vi "生成报告.vi"(6 "目标温度":string(combo), 7 "样品编号":string, 8 "均匀性表格":string[][](table)=[["A", "O", "E", "O"], ["", "", "", ""], ["", "", "", ""], ["", "", "", ""], ["", "", "", ""], ["", "", "", ""], ["", "", "", ""], ["B", "O", "F", "O"], ["", "", "", ""], ["", "", "", ""], ["", "", "", ""], ["", "", "", ""], ["", "", "", ""], ["", "", "", ""], ["C", "O", "G", "O"], ["", "", "", ""], ["", "", "", ""], ["", "", "", ""], ["", "", "", ""], ["", "", "", ""], ["", "", "", ""], ["D", "O", "H", "O"], ["", "", "", ""], ["", "", "", ""], ["", "", "", ""], ["", "", "", ""], ["", "", "", ""], ["", "", "", ""], ["", "", "", ""], ["", "", "", ""]], 10 "波动性表格":string[][](table), 11 "原始记录路径":path caption="模板（空）") -> ()   [LabVIEW 2015]
uses:
  <vilib>/addons/_office/_exclsub.llb/font.ctl
  <vilib>/addons/_office/excel.llb/Excel Easy Table (str).vi
  <vilib>/Utility/NIReport.llb/NI_report.lvclass
  <vilib>/addons/_office/NI_ReportGenerationToolkit.lvlib
  <vilib>/Utility/NIReport.llb/Excel/NI_Excel.lvclass
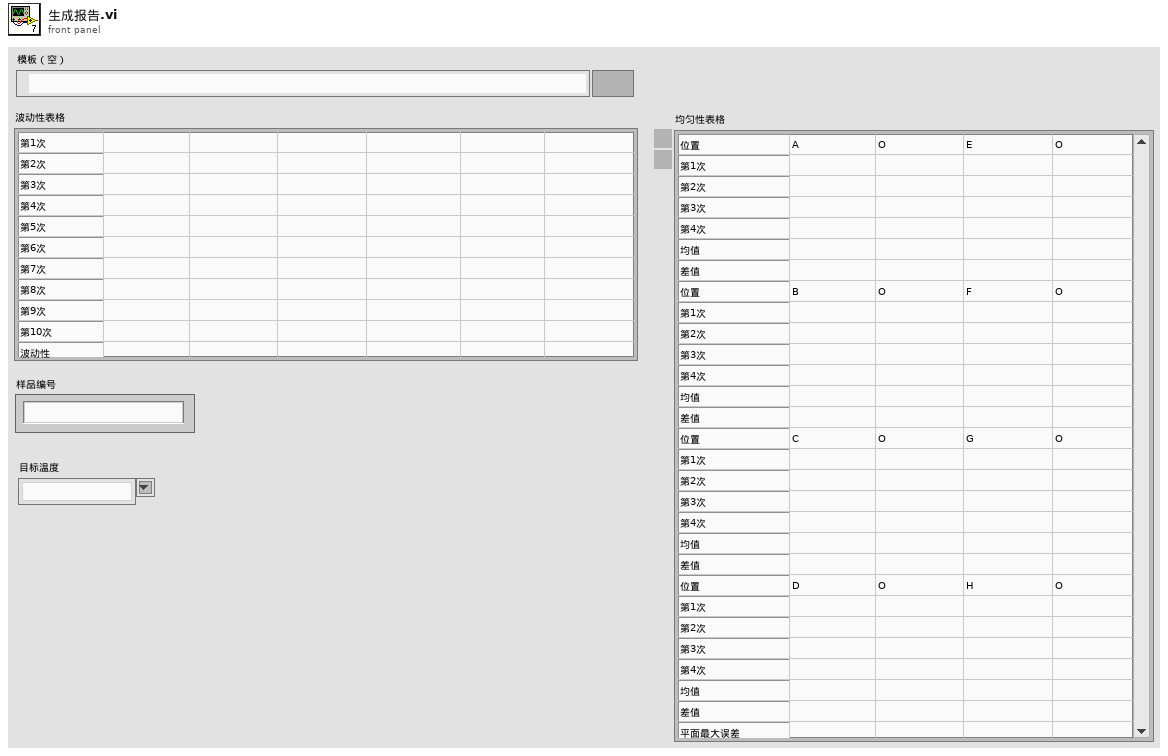
[diagram p1: front panel]
types:
  T1 = typedef "NI_ReportGenerationToolkit.lvlib/font.ctl" = cluster{"font name":string, "font size":dbl, "bold":u16, "italic":u16, "underline":u16, "strike through":u16, "font color":u32}
  T2 = enum16{"maximized", "minimized", "normal", "no change"}
  T3 = enum16{"Standard Report", "HTML", "Word", "Excel"}
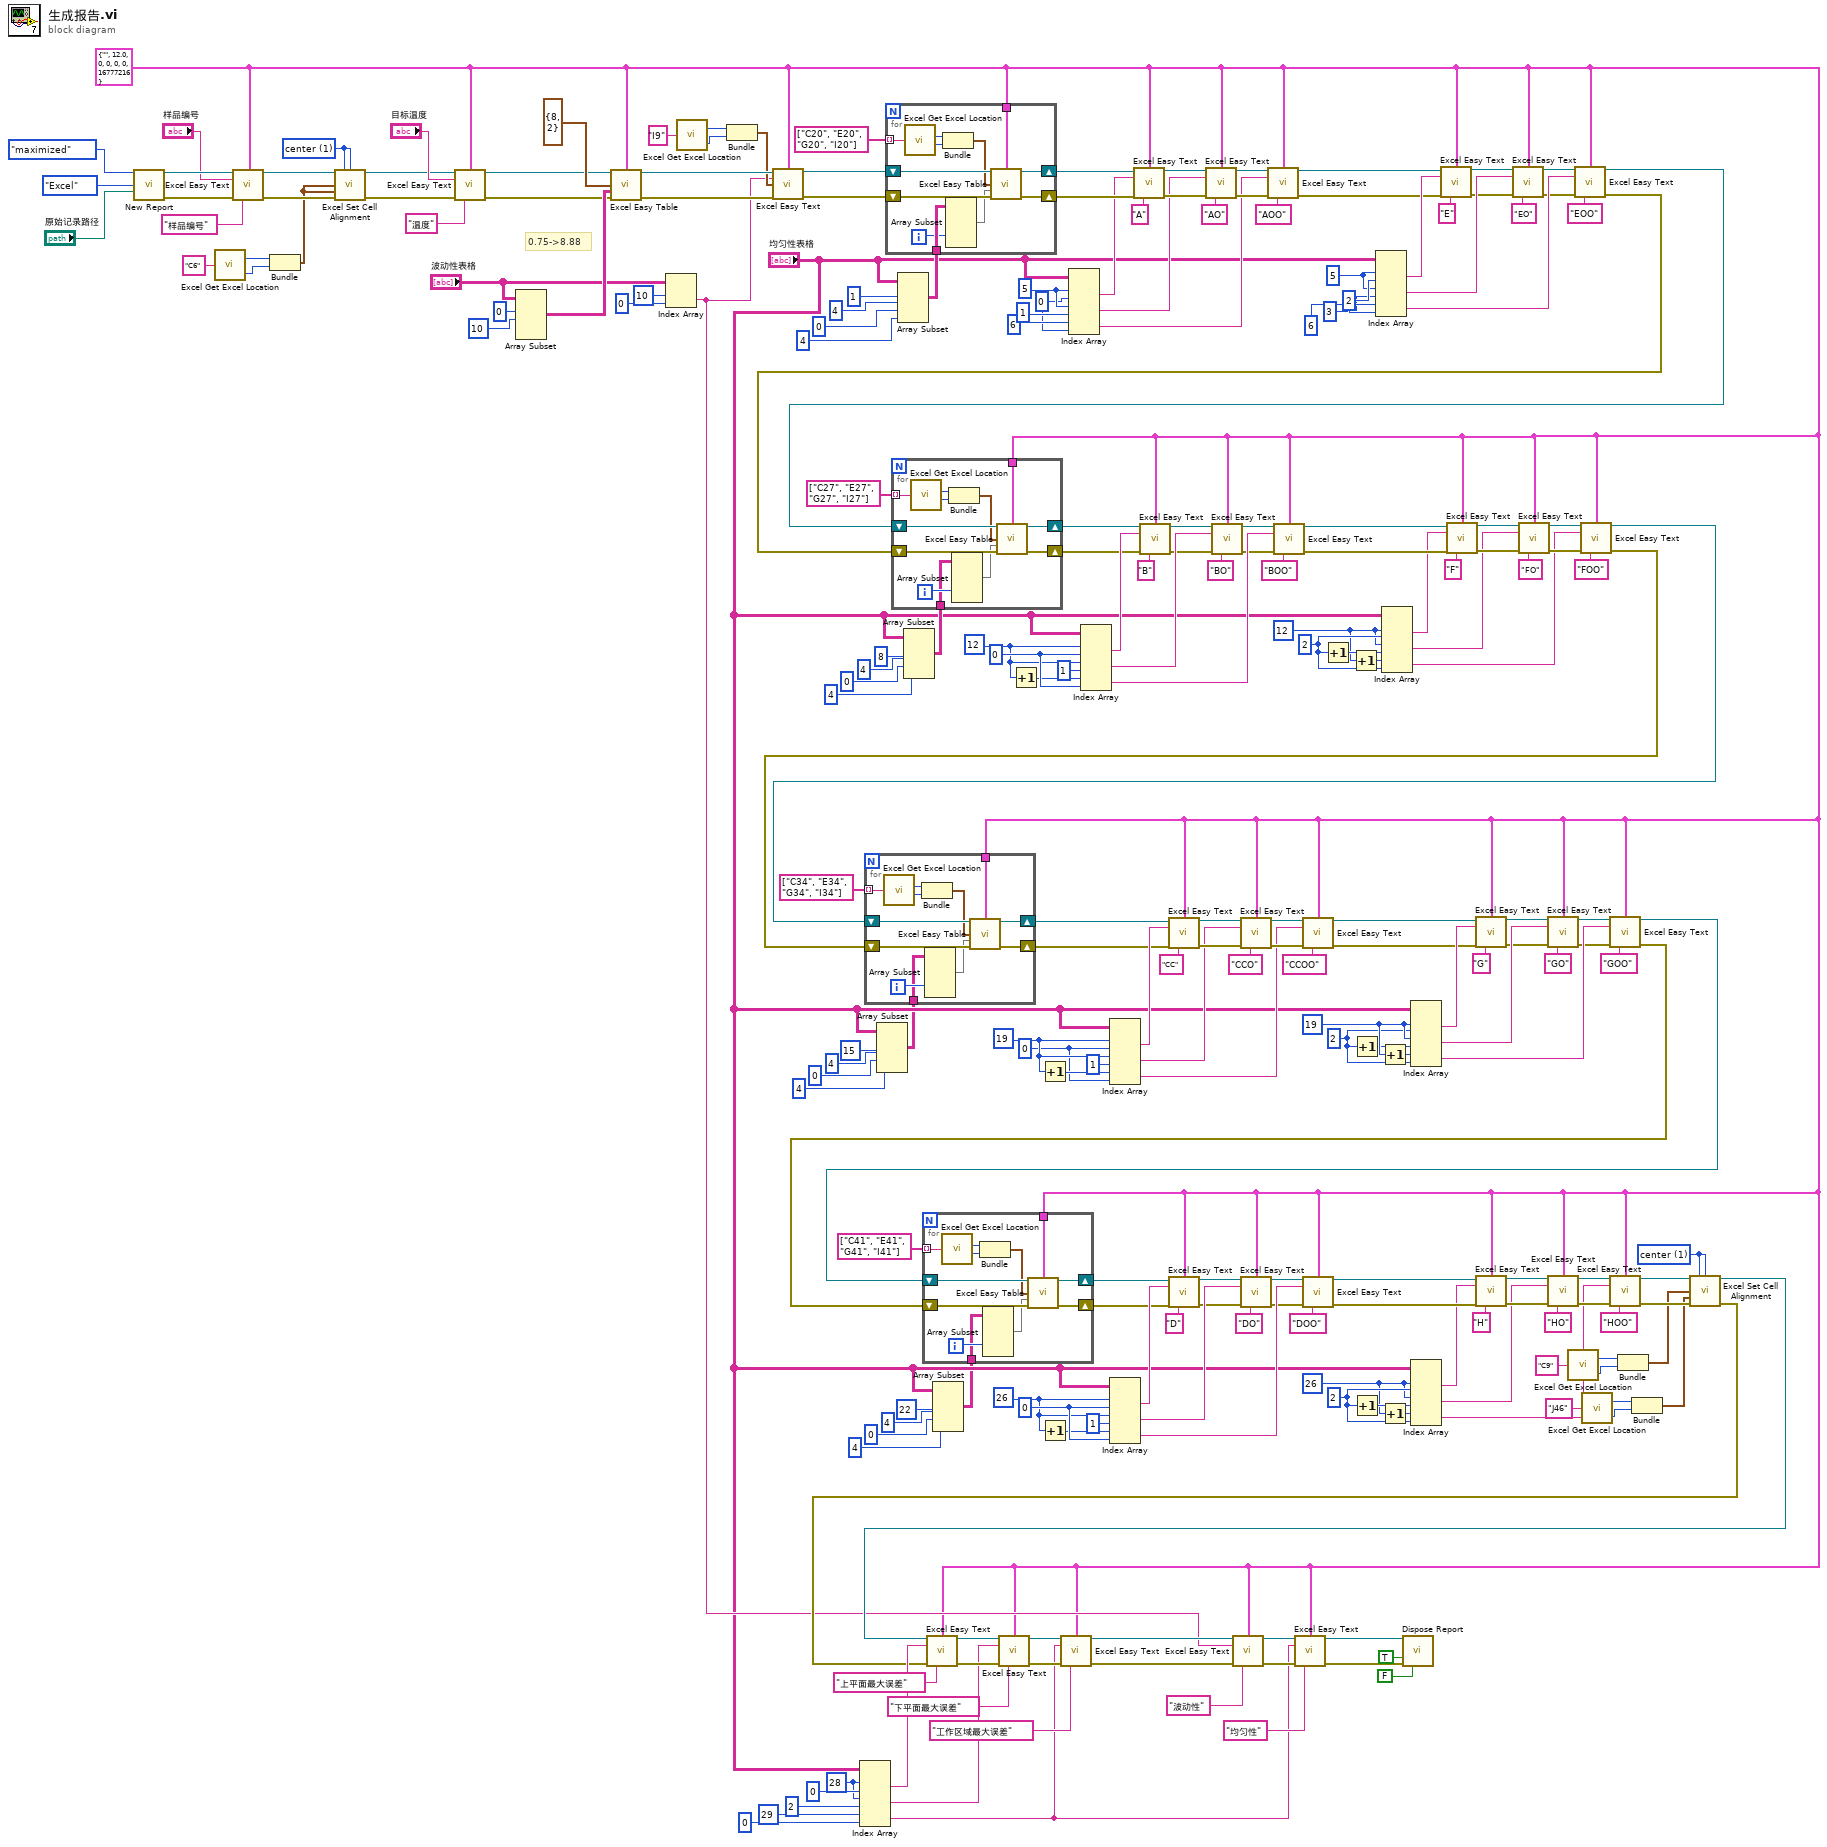
[diagram p0: block diagram]
diagram:
  w30 = 1 items=["top", "center", "bottom"] ("vertical alignment (top)")
  w59 = 1 items=["top", "center", "bottom"] ("vertical alignment (top)")
  w68 = 28 ("索引")
  w81 = 2 ("索引")
  w79 = 26 ("长度")
  w99 = 0 ("索引")
  w83 = 26 ("长度")
  w142 = 2 ("索引")
  w144 = 19 ("长度")
  w124 = 0 ("索引")
  w140 = 19 ("长度")
  w149 = 2 ("索引")
  w147 = 12 ("长度")
  w167 = 0 ("索引")
  w151 = 12 ("长度")
  w3 = T1 {"font name"="", "font size"=12.0, "bold"=0, "italic"=0, "underline"=0, "strike through"=0, "font color"=16777216} ("font")
  w195 = 2 ("索引")
  w192 = 5 ("长度")
  w196 = 0 ("索引")
  w199 = 5 ("长度")
  # "0.75->8.88"
  n1 = call <vilib>:"New Report.vi"("window state (normal)"=T2."maximized", "report type"=T3."Excel", "template (empty)"="原始记录路径") -> ("report out"=w37:refnum<class "NI_report.lvclass">, "error out"=w38:errorcluster)  [unwired: 11 in]
  n2 = call <vilib>:"Excel Get Excel Location.vi"("cell's name"="C6") -> ("row"=w23:i32, "column"=w24:i32)
  n3 = call <vilib>:"Excel Easy Text.vi"("report in"=w37, "font"=w3, "text"="样品编号", "error in (no error)"=w38, "name (\"\")"="样品编号" ("name (\"\")")) -> ("report out"=w27:refnum<class "NI_report.lvclass">, "error out"=w29:errorcluster)  [unwired: 6 in, 3 out]
  n4 = Bundle("row"=w23, "column"=w24) -> (w22:cluster{"row":i32, "column":i32})  [unwired: 1 in]
  n5 = call <vilib>:"Excel Set Cell Alignment.vi"("report in"=w27, "vertical alignment (top)"=w30, "horizontal alignment (left)"=w30, "start (-1, -1)"=w22, "end (-1, -1)"=w22, "error in (no error)"=w29) -> ("report out"=w26:refnum<class "NI_report.lvclass">, "error out"=w28:errorcluster)  [unwired: 8 in]
  n6 = call <vilib>:"Excel Easy Text.vi"("report in"=w26, "font"=w3, "text"="目标温度", "error in (no error)"=w28, "name (\"\")"="温度" ("name (\"\")")) -> ("report out"=w35:refnum<class "NI_report.lvclass">, "error out"=w36:errorcluster)  [unwired: 6 in, 3 out]
  n7 = Array Subset(array="波动性表格", index (row)=0 ("索引"), length (row)=10 ("索引")) -> (w228:string[][])  [unwired: 2 in]
  n8 = call-poly <vilib>:"Excel Easy Table.vi"("report in"=w35, "font"=w3, "start (0, 0)"=cluster{"row":i32, "column":i32} {"row"=8, "column"=2}, "text data"=w228, "error in (no error)"=w36) -> ("report out"=w224:refnum<class "NI_report.lvclass">, "error out"=w223:errorcluster)  [unwired: 6 in, 3 out]
  n9 = Index Array(array="波动性表格", index (row)=10 ("索引 (行)"), index (col)=0 ("索引 (行)")) -> (element=w43:string)
  n10 = call <vilib>:"Excel Get Excel Location.vi"("cell's name"="I9") -> ("row"=w220:i32, "column"=w221:i32)
  n11 = Bundle("row"=w220, "column"=w221) -> (w219:cluster{"row":i32, "column":i32})  [unwired: 1 in]
  n12 = call <vilib>:"Excel Easy Text.vi"("report in"=w224, "font"=w3, "text"=w43, "start (-1, -1)"=w219, "error in (no error)"=w223) -> ("report out"=w218:refnum<class "NI_report.lvclass">, "error out"=w217:errorcluster)  [unwired: 6 in, 3 out]
  n13 = Index Array(array="均匀性表格", index (row) #1=w68, index (col) #1=0 ("索引"), index (row) #2=w68, index (col) #2=2 ("长度"), index (row) #3=29 ("索引"), index (col) #3=0 ("索引")) -> (element #1=w70:string, element #2=w64:string, element #3=w44:string)
  n14 = Array Subset(array="均匀性表格", index (row)=15 ("索引"), length (row)=4 ("长度"), index (col)=0 ("索引"), length (col)=4 ("索引")) -> (w1:string[][])
  n15 = Array Subset(array="均匀性表格", index (row)=1 ("索引"), length (row)=4 ("长度"), index (col)=0 ("索引"), length (col)=4 ("索引")) -> (w212:string[][])
  n16 = for {
    tunnel: w212 -> [w237]
    tunnel: w3 -> [w239]
    shift-right: [w240] -> w210
    shift-left: w218 -> [w246]
    shift-right: [w241] -> w211
    shift-left: w217 -> [w245]
    tunnel: string[] ["C20", "E20", "G20", "I20"] -> [w238] mode=indexing
    i -> [w235]
    n17 = call <vilib>:"Excel Get Excel Location.vi"("cell's name"=w238) -> ("row"=w244:i32, "column"=w243:i32)
    n18 = Bundle("row"=w244, "column"=w243) -> (w242:cluster{"row":i32, "column":i32})  [unwired: 1 in]
    n19 = Array Subset(array=w237, index (col)=w235) -> (w236:string[][])  [unwired: 3 in]
    n20 = call-poly <vilib>:"Excel Easy Table.vi"("report in"=w246, "font"=w239, "start (0, 0)"=w242, "text data"=w236, "error in (no error)"=w245) -> ("report out"=w240:refnum<class "NI_report.lvclass">, "error out"=w241:errorcluster)  [unwired: 6 in, 3 out]
  }
  n21 = Array Subset(array="均匀性表格", index (row)=8 ("索引"), length (row)=4 ("长度"), index (col)=0 ("索引"), length (col)=4 ("索引")) -> (w15:string[][])
  n22 = Array Subset(array="均匀性表格", index (row)=22 ("索引"), length (row)=4 ("长度"), index (col)=0 ("索引"), length (col)=4 ("索引")) -> (w2:string[][])
  n23 = Increment(x=w151) -> (x+1=w150:i32)
  n24 = Increment(x=w140) -> (x+1=w141:i32)
  n25 = Increment(x=w83) -> (x+1=w82:i32)
  n26 = Index Array(array="均匀性表格", index (row) #1=w199, index (col) #1=w196, index (row) #2=w199, index (col) #2=1 ("索引"), index (row) #3=6 ("长度"), index (col) #3=w196) -> (element #1=w209:string, element #2=w201:string, element #3=w200:string)
  n27 = Index Array(array="均匀性表格", index (row) #1=w151, index (col) #1=w167, index (row) #2=w151, index (col) #2=1 ("索引"), index (row) #3=w150, index (col) #3=w167) -> (element #1=w156:string, element #2=w164:string, element #3=w165:string)
  n28 = Index Array(array="均匀性表格", index (row) #1=w140, index (col) #1=w124, index (row) #2=w140, index (col) #2=1 ("索引"), index (row) #3=w141, index (col) #3=w124) -> (element #1=w135:string, element #2=w127:string, element #3=w126:string)
  n29 = Index Array(array="均匀性表格", index (row) #1=w83, index (col) #1=w99, index (row) #2=w83, index (col) #2=1 ("索引"), index (row) #3=w82, index (col) #3=w99) -> (element #1=w88:string, element #2=w96:string, element #3=w97:string)
  n30 = call <vilib>:"Excel Easy Text.vi"("report in"=w210, "font"=w3, "text"=w209, "error in (no error)"=w211, "name (\"\")"="A" ("name (\"\")")) -> ("report out"=w207:refnum<class "NI_report.lvclass">, "error out"=w206:errorcluster)  [unwired: 6 in, 3 out]
  n31 = call <vilib>:"Excel Easy Text.vi"("report in"=w207, "font"=w3, "text"=w201, "error in (no error)"=w206, "name (\"\")"="AO" ("name (\"\")")) -> ("report out"=w203:refnum<class "NI_report.lvclass">, "error out"=w202:errorcluster)  [unwired: 6 in, 3 out]
  n32 = call <vilib>:"Excel Easy Text.vi"("report in"=w203, "font"=w3, "text"=w200, "error in (no error)"=w202, "name (\"\")"="AOO" ("name (\"\")")) -> ("report out"=w180:refnum<class "NI_report.lvclass">, "error out"=w181:errorcluster)  [unwired: 6 in, 3 out]
  n33 = Increment(x=w149) -> (x+1=w148:i32)
  n34 = Increment(x=w147) -> (x+1=w146:i32)
  n35 = Increment(x=w142) -> (x+1=w143:i32)
  n36 = Increment(x=w81) -> (x+1=w80:i32)
  n37 = Index Array(array="均匀性表格", index (row) #1=w192, index (col) #1=w195, index (row) #2=w192, index (col) #2=3 ("索引"), index (row) #3=6 ("长度"), index (col) #3=w195) -> (element #1=w182:string, element #2=w190:string, element #3=w191:string)
  n38 = Increment(x=w144) -> (x+1=w145:i32)
  n39 = Increment(x=w79) -> (x+1=w78:i32)
  n40 = Index Array(array="均匀性表格", index (row) #1=w147, index (col) #1=w149, index (row) #2=w147, index (col) #2=w148, index (row) #3=w146, index (col) #3=w149) -> (element #1=w177:string, element #2=w169:string, element #3=w168:string)
  n41 = Index Array(array="均匀性表格", index (row) #1=w144, index (col) #1=w142, index (row) #2=w144, index (col) #2=w143, index (row) #3=w145, index (col) #3=w142) -> (element #1=w114:string, element #2=w122:string, element #3=w123:string)
  n42 = Index Array(array="均匀性表格", index (row) #1=w79, index (col) #1=w81, index (row) #2=w79, index (col) #2=w80, index (row) #3=w78, index (col) #3=w81) -> (element #1=w109:string, element #2=w101:string, element #3=w100:string)
  n43 = call <vilib>:"Excel Easy Text.vi"("report in"=w180, "font"=w3, "text"=w182, "error in (no error)"=w181, "name (\"\")"="E" ("name (\"\")")) -> ("report out"=w184:refnum<class "NI_report.lvclass">, "error out"=w185:errorcluster)  [unwired: 6 in, 3 out]
  n44 = call <vilib>:"Excel Easy Text.vi"("report in"=w184, "font"=w3, "text"=w190, "error in (no error)"=w185, "name (\"\")"="EO" ("name (\"\")")) -> ("report out"=w188:refnum<class "NI_report.lvclass">, "error out"=w189:errorcluster)  [unwired: 6 in, 3 out]
  n45 = call <vilib>:"Excel Get Excel Location.vi"("cell's name"="C9") -> ("row"=w56:i32, "column"=w57:i32)
  n46 = call <vilib>:"Excel Easy Text.vi"("report in"=w188, "font"=w3, "text"=w191, "error in (no error)"=w189, "name (\"\")"="EOO" ("name (\"\")")) -> ("report out"=w20:refnum<class "NI_report.lvclass">, "error out"=w19:errorcluster)  [unwired: 6 in, 3 out]
  n47 = for {
    tunnel: w15 -> [w247]
    tunnel: w3 -> [w251]
    shift-right: [w252] -> w18
    shift-left: w20 -> [w258]
    shift-right: [w253] -> w17
    shift-left: w19 -> [w257]
    tunnel: string[] ["C27", "E27", "G27", "I27"] -> [w250] mode=indexing
    i -> [w248]
    n48 = call <vilib>:"Excel Get Excel Location.vi"("cell's name"=w250) -> ("row"=w256:i32, "column"=w255:i32)
    n49 = Bundle("row"=w256, "column"=w255) -> (w254:cluster{"row":i32, "column":i32})  [unwired: 1 in]
    n50 = Array Subset(array=w247, index (col)=w248) -> (w249:string[][])  [unwired: 3 in]
    n51 = call-poly <vilib>:"Excel Easy Table.vi"("report in"=w258, "font"=w251, "start (0, 0)"=w254, "text data"=w249, "error in (no error)"=w257) -> ("report out"=w252:refnum<class "NI_report.lvclass">, "error out"=w253:errorcluster)  [unwired: 6 in, 3 out]
  }
  n52 = call <vilib>:"Excel Easy Text.vi"("report in"=w18, "font"=w3, "text"=w156, "error in (no error)"=w17, "name (\"\")"="B" ("name (\"\")")) -> ("report out"=w158:refnum<class "NI_report.lvclass">, "error out"=w159:errorcluster)  [unwired: 6 in, 3 out]
  n53 = call <vilib>:"Excel Easy Text.vi"("report in"=w158, "font"=w3, "text"=w164, "error in (no error)"=w159, "name (\"\")"="BO" ("name (\"\")")) -> ("report out"=w162:refnum<class "NI_report.lvclass">, "error out"=w163:errorcluster)  [unwired: 6 in, 3 out]
  n54 = call <vilib>:"Excel Easy Text.vi"("report in"=w162, "font"=w3, "text"=w165, "error in (no error)"=w163, "name (\"\")"="BOO" ("name (\"\")")) -> ("report out"=w179:refnum<class "NI_report.lvclass">, "error out"=w178:errorcluster)  [unwired: 6 in, 3 out]
  n55 = call <vilib>:"Excel Easy Text.vi"("report in"=w179, "font"=w3, "text"=w177, "error in (no error)"=w178, "name (\"\")"="F" ("name (\"\")")) -> ("report out"=w175:refnum<class "NI_report.lvclass">, "error out"=w174:errorcluster)  [unwired: 6 in, 3 out]
  n56 = call <vilib>:"Excel Easy Text.vi"("report in"=w175, "font"=w3, "text"=w169, "error in (no error)"=w174, "name (\"\")"="FO" ("name (\"\")")) -> ("report out"=w171:refnum<class "NI_report.lvclass">, "error out"=w170:errorcluster)  [unwired: 6 in, 3 out]
  n57 = call <vilib>:"Excel Easy Text.vi"("report in"=w171, "font"=w3, "text"=w168, "error in (no error)"=w170, "name (\"\")"="FOO" ("name (\"\")")) -> ("report out"=w10:refnum<class "NI_report.lvclass">, "error out"=w9:errorcluster)  [unwired: 6 in, 3 out]
  n58 = for {
    tunnel: w1 -> [w259]
    tunnel: w3 -> [w263]
    shift-right: [w264] -> w12
    shift-left: w10 -> [w270]
    shift-right: [w265] -> w13
    shift-left: w9 -> [w269]
    tunnel: string[] ["C34", "E34", "G34", "I34"] -> [w262] mode=indexing
    i -> [w260]
    n59 = call <vilib>:"Excel Get Excel Location.vi"("cell's name"=w262) -> ("row"=w268:i32, "column"=w267:i32)
    n60 = Bundle("row"=w268, "column"=w267) -> (w266:cluster{"row":i32, "column":i32})  [unwired: 1 in]
    n61 = Array Subset(array=w259, index (col)=w260) -> (w261:string[][])  [unwired: 3 in]
    n62 = call-poly <vilib>:"Excel Easy Table.vi"("report in"=w270, "font"=w263, "start (0, 0)"=w266, "text data"=w261, "error in (no error)"=w269) -> ("report out"=w264:refnum<class "NI_report.lvclass">, "error out"=w265:errorcluster)  [unwired: 6 in, 3 out]
  }
  n63 = call <vilib>:"Excel Easy Text.vi"("report in"=w12, "font"=w3, "text"=w135, "error in (no error)"=w13, "name (\"\")"="CC" ("name (\"\")")) -> ("report out"=w133:refnum<class "NI_report.lvclass">, "error out"=w132:errorcluster)  [unwired: 6 in, 3 out]
  n64 = call <vilib>:"Excel Easy Text.vi"("report in"=w133, "font"=w3, "text"=w127, "error in (no error)"=w132, "name (\"\")"="CCO" ("name (\"\")")) -> ("report out"=w129:refnum<class "NI_report.lvclass">, "error out"=w128:errorcluster)  [unwired: 6 in, 3 out]
  n65 = call <vilib>:"Excel Easy Text.vi"("report in"=w129, "font"=w3, "text"=w126, "error in (no error)"=w128, "name (\"\")"="CCOO" ("name (\"\")")) -> ("report out"=w112:refnum<class "NI_report.lvclass">, "error out"=w113:errorcluster)  [unwired: 6 in, 3 out]
  n66 = call <vilib>:"Excel Easy Text.vi"("report in"=w112, "font"=w3, "text"=w114, "error in (no error)"=w113, "name (\"\")"="G" ("name (\"\")")) -> ("report out"=w116:refnum<class "NI_report.lvclass">, "error out"=w117:errorcluster)  [unwired: 6 in, 3 out]
  n67 = call <vilib>:"Excel Easy Text.vi"("report in"=w116, "font"=w3, "text"=w122, "error in (no error)"=w117, "name (\"\")"="GO" ("name (\"\")")) -> ("report out"=w120:refnum<class "NI_report.lvclass">, "error out"=w121:errorcluster)  [unwired: 6 in, 3 out]
  n68 = call <vilib>:"Excel Get Excel Location.vi"("cell's name"="J46") -> ("row"=w55:i32, "column"=w54:i32)
  n69 = call <vilib>:"Excel Easy Text.vi"("report in"=w120, "font"=w3, "text"=w123, "error in (no error)"=w121, "name (\"\")"="GOO" ("name (\"\")")) -> ("report out"=w5:refnum<class "NI_report.lvclass">, "error out"=w4:errorcluster)  [unwired: 6 in, 3 out]
  n70 = for {
    tunnel: w2 -> [w271]
    tunnel: w3 -> [w275]
    shift-right: [w276] -> w7
    shift-left: w5 -> [w282]
    shift-right: [w277] -> w6
    shift-left: w4 -> [w281]
    tunnel: string[] ["C41", "E41", "G41", "I41"] -> [w274] mode=indexing
    i -> [w272]
    n71 = call <vilib>:"Excel Get Excel Location.vi"("cell's name"=w274) -> ("row"=w280:i32, "column"=w279:i32)
    n72 = Bundle("row"=w280, "column"=w279) -> (w278:cluster{"row":i32, "column":i32})  [unwired: 1 in]
    n73 = Array Subset(array=w271, index (col)=w272) -> (w273:string[][])  [unwired: 3 in]
    n74 = call-poly <vilib>:"Excel Easy Table.vi"("report in"=w282, "font"=w275, "start (0, 0)"=w278, "text data"=w273, "error in (no error)"=w281) -> ("report out"=w276:refnum<class "NI_report.lvclass">, "error out"=w277:errorcluster)  [unwired: 6 in, 3 out]
  }
  n75 = call <vilib>:"Excel Easy Text.vi"("report in"=w7, "font"=w3, "text"=w88, "error in (no error)"=w6, "name (\"\")"="D" ("name (\"\")")) -> ("report out"=w90:refnum<class "NI_report.lvclass">, "error out"=w91:errorcluster)  [unwired: 6 in, 3 out]
  n76 = call <vilib>:"Excel Easy Text.vi"("report in"=w90, "font"=w3, "text"=w96, "error in (no error)"=w91, "name (\"\")"="DO" ("name (\"\")")) -> ("report out"=w94:refnum<class "NI_report.lvclass">, "error out"=w95:errorcluster)  [unwired: 6 in, 3 out]
  n77 = call <vilib>:"Excel Easy Text.vi"("report in"=w94, "font"=w3, "text"=w97, "error in (no error)"=w95, "name (\"\")"="DOO" ("name (\"\")")) -> ("report out"=w111:refnum<class "NI_report.lvclass">, "error out"=w110:errorcluster)  [unwired: 6 in, 3 out]
  n78 = call <vilib>:"Excel Easy Text.vi"("report in"=w111, "font"=w3, "text"=w109, "error in (no error)"=w110, "name (\"\")"="H" ("name (\"\")")) -> ("report out"=w107:refnum<class "NI_report.lvclass">, "error out"=w106:errorcluster)  [unwired: 6 in, 3 out]
  n79 = call <vilib>:"Excel Easy Text.vi"("report in"=w107, "font"=w3, "text"=w101, "error in (no error)"=w106, "name (\"\")"="HO" ("name (\"\")")) -> ("report out"=w103:refnum<class "NI_report.lvclass">, "error out"=w102:errorcluster)  [unwired: 6 in, 3 out]
  n80 = call <vilib>:"Excel Easy Text.vi"("report in"=w103, "font"=w3, "text"=w100, "error in (no error)"=w102, "name (\"\")"="HOO" ("name (\"\")")) -> ("report out"=w63:refnum<class "NI_report.lvclass">, "error out"=w61:errorcluster)  [unwired: 6 in, 3 out]
  n81 = Bundle("row"=w56, "column"=w57) -> (w52:cluster{"row":i32, "column":i32})  [unwired: 1 in]
  n82 = Bundle("row"=w55, "column"=w54) -> (w51:cluster{"row":i32, "column":i32})  [unwired: 1 in]
  n83 = call <vilib>:"Excel Set Cell Alignment.vi"("report in"=w63, "vertical alignment (top)"=w59, "horizontal alignment (left)"=w59, "start (-1, -1)"=w52, "end (-1, -1)"=w51, "error in (no error)"=w61) -> ("report out"=w62:refnum<class "NI_report.lvclass">, "error out"=w60:errorcluster)  [unwired: 8 in]
  n84 = call <vilib>:"Excel Easy Text.vi"("report in"=w62, "font"=w3, "text"=w70, "error in (no error)"=w60, "name (\"\")"="上平面最大误差" ("name (\"\")")) -> ("report out"=w72:refnum<class "NI_report.lvclass">, "error out"=w73:errorcluster)  [unwired: 6 in, 3 out]
  n85 = call <vilib>:"Excel Easy Text.vi"("report in"=w72, "font"=w3, "text"=w64, "error in (no error)"=w73, "name (\"\")"="下平面最大误差" ("name (\"\")")) -> ("report out"=w76:refnum<class "NI_report.lvclass">, "error out"=w77:errorcluster)  [unwired: 6 in, 3 out]
  n86 = call <vilib>:"Excel Easy Text.vi"("report in"=w76, "font"=w3, "text"=w44, "error in (no error)"=w77, "name (\"\")"="工作区域最大误差" ("name (\"\")")) -> ("report out"=w47:refnum<class "NI_report.lvclass">, "error out"=w46:errorcluster)  [unwired: 6 in, 3 out]
  n87 = call <vilib>:"Excel Easy Text.vi"("report in"=w47, "font"=w3, "text"=w43, "error in (no error)"=w46, "name (\"\")"="波动性" ("name (\"\")")) -> ("report out"=w49:refnum<class "NI_report.lvclass">, "error out"=w48:errorcluster)  [unwired: 6 in, 3 out]
  n88 = call <vilib>:"Excel Easy Text.vi"("report in"=w49, "font"=w3, "text"=w44, "error in (no error)"=w48, "name (\"\")"="均匀性" ("name (\"\")")) -> ("report out"=w42:refnum<class "NI_report.lvclass">, "error out"=w41:errorcluster)  [unwired: 6 in, 3 out]
  n89 = call-dynamic "Dispose Report.vi"("report in"=w42, "save changes? (F)"=TRUE, "error in (no error)"=w41, "close report? (T)"=FALSE) -> ()  [unwired: 11 in, 1 out]
